vi "Creators Created Events.vi"(8 "Created Event Alias":string, 9 "Priority?":bool, 10 "Msg Strategy":refnum<class "Msg Strategy.lvclass">, 11 "eeeee in":refnum<class "eeeee.lvclass">) -> (3 "eeeee out":refnum<class "eeeee.lvclass">)   [LabVIEW 2021, in "Providers.lvlib" / "eeeee.lvlib" / "eeeee.lvclass"]
uses:
  jettl/Msg Strategy/Msg Strategy.lvclass
  eeeee.lvclass
  eeeee.lvclass/eeeee.ctl
  jettl/Event/Event.lvclass
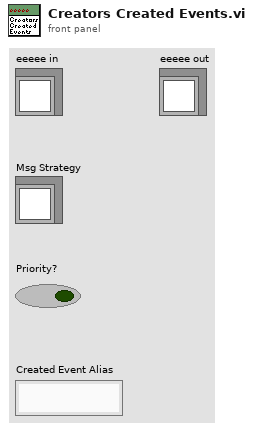
[diagram p1: front panel]
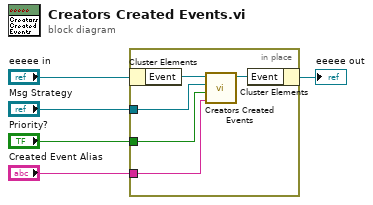
[diagram p0: block diagram]
diagram:
  n1 = in-place {
    in-place-border: "Msg Strategy" -> [w8]
    in-place-border: "Priority?" -> [w7]
    in-place-border: "Created Event Alias" -> [w6]
    n2 = in-place-cluster #1("eeeee in") -> ("Event"=w10:refnum<class "Event.lvclass">)
    n3 = call-dynamic "Creators Created Events.vi"("Created Event Alias"=w6, "Priority?"=w7, "Msg Strategy"=w8, "Event in"=w10) -> ("Event out"=w9:refnum<class "Event.lvclass">)  [unwired: 7 in]
    n4 = in-place-cluster #1("Event"=w9) -> (→"eeeee out":refnum<class "eeeee.lvclass">)
  }
